vi "Details Display Dialog-MOD.vi"(0 "Source":string, 1 "Start":i32[](array[numeric]), 2 "Length":i32[](array[numeric]), 5 "Details":string="reason for problem", 7 "dialog type":T2, 9 "Error or Warning":bool, 11 "contname":string="Continue", 12 "stopname":string="Stop", 13 "okname":string="OK") -> (4 "STOP?":bool, 15 "stop event propagated":bool)   [LabVIEW 2013]
uses:
  <vilib>/Utility/error.llb/DialogTypeEnum.ctl
  <vilib>/Utility/error.llb/ErrWarn.ctl
  <vilib>/event_ctls.llb/eventvkey.ctl
panel:
  in  "truncated message":string="(source truncated)"
  in  "truncated & CH message":string="(source truncated; see Context Help window)"
  out "Source of Error":string
  out "scrollbar text":string
  in  "Test for size":string
  out "text":string
  out "Error or Warning Glyph":T1=TRUE
  in  "OK":bool
  in  "Stop":bool
  in  "Continue":bool
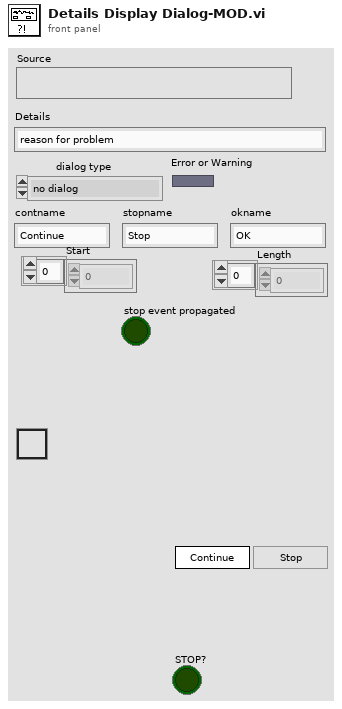
[diagram p1: front panel]
types:
  T1 = typedef "ErrWarn.ctl" = bool
  T2 = typedef "DialogTypeEnum.ctl" = enum16{"no dialog", "OK message", "continue or stop message", "auto error handling dialog", "OK message + warnings", "continue/stop + warnings"}
  T3 = typedef "eventvkey.ctl" = enum16{"ASCII", "Enter", "Return", "Shift", "Ctrl", "Alt", "Cmd", "Opt", "Caps", "NumLock", "Clear", "Break", "Up", "Down", "Left", "Right", "Insert", "Delete", "Home", "End", "PageUp", "PageDown", "Escape", "Help", "Pause", "ScrollLock", "F1", "F2", "F3", "F4", "F5", "F6", "F7", "F8", "F9", "F10", "F11", "F12", "F13", "F14", "F15", "F16", "F17", "F18", "F19", "F20", "F21", "F22", "F23", "F24", "Play", "VolumeUp", "VolumeDown", "Mute", "Two Byte Char"}
  T4 = typedef "LVRectTypeDef.ctl" = cluster{"Left":i16, "Top":i16, "Right":i16, "Bottom":i16}
  T5 = cluster{"Control":bool, "Shift":bool, "Key":string}
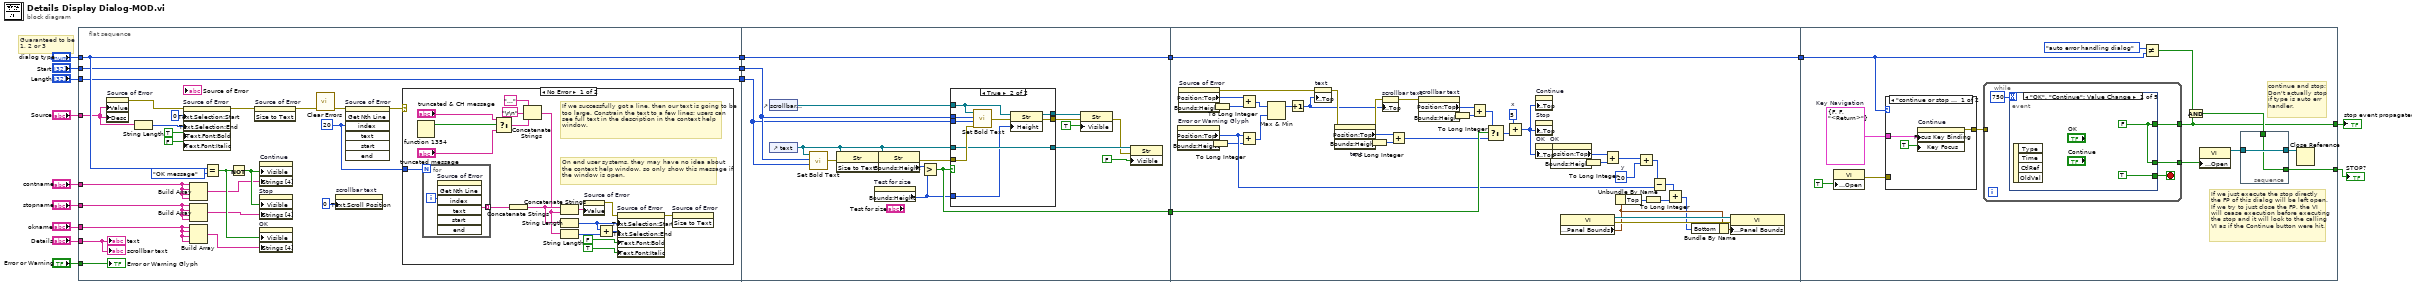
[diagram p0: block diagram]
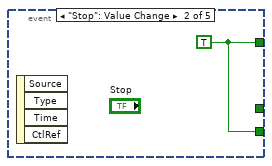
[diagram p4: hidden frame]
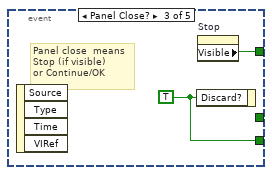
[diagram p5: hidden frame]
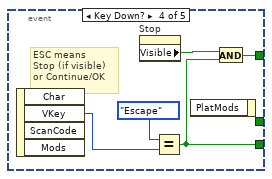
[diagram p6: hidden frame]
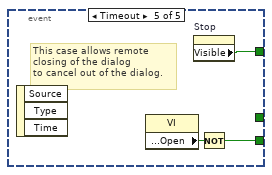
[diagram p7: hidden frame]
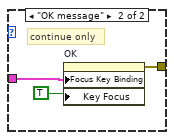
[diagram p8: hidden frame]
diagram:
  # "Guaranteed to be\n1, 2 or 3"
  n1 = flat-sequence {
    tunnel: [w26] -> w16
    tunnel: "dialog type" -> [w26]
    tunnel: "contname" -> [w25]
    tunnel: "stopname" -> [w24]
    tunnel: "okname" -> [w23]
    tunnel: "Source" -> [w18]
    tunnel: "Details" -> [w22]
    tunnel: "Error or Warning" -> [w21]
    tunnel: [w20] -> w5
    tunnel: [w19] -> w4
    tunnel: "Start" -> [w20]
    tunnel: "Length" -> [w19]
    tunnel: w16 -> [w66]
    tunnel: [w66] -> w15
    tunnel: [w72] -> w14
    tunnel: w5 -> [w65]
    tunnel: w4 -> [w64]
    tunnel: w15 -> [w99]
    tunnel: [w99] -> w13
    tunnel: w14 -> [w134]
    tunnel: [w136] -> w17
    tunnel: w13 -> [w138]
    tunnel: [w135] -> w1
    frame #0 {
      w33 = u32 20 ("index")
      n2 = property on="Source of Error" class="Str"("Value"=w18, "Desc"=w18) -> (error out=w32:errorcluster)  [unwired: 2 in, 1 out]
      n3 = String Length(string=w18) -> (length=w29:i32)
      n4 = property on="Source of Error" class="Str"(error in=w32, "Text.Selection:Start"=u32 0, "Text.Selection:End"=w29, "Text.Font:Bold"=TRUE, "Text.Font:Italic"=FALSE) -> (error out=w31:errorcluster)  [unwired: 1 in, 1 out]
      n5 = Build Array(w25, w25, w25, w25) -> (w41:string[])
      n6 = Build Array(w24, w24, w24, w24) -> (w40:string[])
      n7 = Build Array(w23, w23, w23, w23) -> (w39:string[])
      n8 = Equal?(x=w26, y=DialogTypeEnum."OK message" ("dialog type")) -> (x = y?=w43:bool)
      n9 = Not(x=w43) -> (.not. x?=w42:bool)
      n10 = invoke on="Source of Error" class="Str" method="Size to Text"(error in=w31) -> (error out=w36:errorcluster)  [unwired: 2 in, 2 out]
      n11 = property on="Continue" class="Bool"("Visible"=w42, "Strings [4]"=w41) -> ()  [unwired: 2 in, 2 out]
      n12 = property on="Stop" class="Bool"("Visible"=w42, "Strings [4]"=w40) -> ()  [unwired: 2 in, 2 out]
      n13 = property on="OK" class="Bool"("Visible"=w43, "Strings [4]"=w39) -> ()  [unwired: 2 in, 2 out]
      n14 = call <vilib>:"Clear Errors.vi"("error in (no error)"=w36) -> ("error out"=w35:errorcluster)  [unwired: 6 out]
      n15 = property on="scrollbar text" class="Str"("Text.Scroll Position"=u32 0) -> ()  [unwired: 2 in, 2 out]
      n16 = invoke on="Source of Error" class="Str" method="Get Nth Line"(error in=w35, "index"=w33) -> (error out=w34:errorcluster)  [unwired: 5 in, 6 out]
      n17 = case shown="No Error" w34 {
        tunnel: w33 -> [w61 _]
        frame No Error {
          # "If we successfully got a line, then our text is going to be too large. Constrain the text to a few lines; users can see full text in the description in the context help window."
          # "On end user systems, they may have no idea about\nthe context help window, so only show this message if\nthe window is open."
          n18 = fn#1354() -> (1:w51:bool)  [unwired: 1 out]
          n19 = for {
            N: w61 -> [_]
            tunnel: [w62] -> w59 mode=indexing
            i -> [w63]
            n20 = invoke on="Source of Error" class="Str" method="Get Nth Line"("index"=w63) -> ("text"=w62:string)  [unwired: 6 in, 6 out]
          }
          n21 = Select(t="truncated & CH message", s=w51, f="truncated message") -> (s? t:f=w48:string)
          n22 = Concatenate Strings(w59) -> (w58:string)
          n23 = Concatenate Strings("..." ("string"), "\r\n", w48) -> (w45:string)
          n24 = Concatenate Strings(w58, w45) -> (w60:string)
          n25 = String Length(string=w58) -> (length=w53:i32)
          n26 = String Length(string=w45) -> (length=w50:i32)
          n27 = property on="Source of Error" class="Str"("Value"=w60) -> (error out=w55:errorcluster)  [unwired: 2 in, 1 out]
          n28 = Add(x=w53, y=w50) -> (x+y=w52:i32)
          n29 = property on="Source of Error" class="Str"(error in=w55, "Text.Selection:Start"=w53, "Text.Selection:End"=w52, "Text.Font:Bold"=FALSE, "Text.Font:Italic"=TRUE) -> (error out=w54:errorcluster)  [unwired: 1 in, 1 out]
          n30 = invoke on="Source of Error" class="Str" method="Size to Text"(error in=w54) -> ()  [unwired: 2 in, 3 out]
        }
        frame Error {
          # "An error at this point means that there is no line to fetch. That's good. We do not want the text getting too large."
        }
      }
      "Error or Warning Glyph" <- w21
      "scrollbar text" <- w22
      "text" <- w22
    }
    frame #1 {
      n31 = control-ref of="scrollbar text"() -> (w75:refnum<vi>)
      n32 = control-ref of="text"() -> (w67:refnum<vi>)
      n33 = call <vilib>:"Set Bold Text.vi"("Length"=w64, "Start"=w65, "text"=w67) -> ("error out"=w70:errorcluster)  [unwired: 1 in, 2 out]
      n34 = invoke class="Str" method="Size to Text"(reference=w67, error in=w70) -> (error out=w71:errorcluster)  [unwired: 1 in, 2 out]
      n35 = property on="Test for size" class="Str"() -> ("Bounds:Height"=w69:u32)  [unwired: 2 in, 2 out]
      n36 = property class="Str"(reference=w67, error in=w71) -> (error out=w79:errorcluster, "Bounds:Height"=w80:u32)  [unwired: 1 out]
      n37 = Greater?(x=w80, y=w69) -> (0:w72:bool)
      n38 = case shown="True" w72 {
        tunnel: w79 -> [w83 w92]
        tunnel: w65 -> [_ w91]
        tunnel: w64 -> [_ w90]
        tunnel: [w83 w87] -> w68
        tunnel: w67 -> [w82 w89]
        tunnel: [w82 w84] -> w77
        tunnel: [w81 w89] -> w76
        tunnel: w75 -> [w81 w85]
        tunnel: w69 -> [_ w88]
        frame False {
        }
        frame True {
          n39 = call <vilib>:"Set Bold Text.vi"("error in"=w92, "Length"=w90, "Start"=w91, "text"=w85) -> ("error out"=w86:errorcluster)  [unwired: 2 out]
          n40 = property class="Str"(reference=w85, error in=w86, "Height"=w88) -> (reference out=w84:refnum<vi>, error out=w87:errorcluster)
        }
      }
      n41 = property class="Str"(reference=w77, error in=w68, "Visible"=TRUE ("Defer Panel Updates")) -> (error out=w73:errorcluster)  [unwired: 1 out]
      n42 = property class="Str"(reference=w76, error in=w73, "Visible"=FALSE ("Defer Panel Updates")) -> ()  [unwired: 2 out]
    }
    frame #2 {
      w120 = 20  # y
      w125 = 5  # x
      n43 = property on="Error or Warning Glyph" class="Bool"() -> ("Position:Top"=w115:i32, "Bounds:Height"=w131:u32)  [unwired: 2 in, 2 out]
      n44 = property on="Source of Error" class="Str"() -> (error out=w100:errorcluster, "Position:Top"=w102:i32, "Bounds:Height"=w101:u32)  [unwired: 2 in, 1 out]
      n45 = To Long Integer(number=w131) -> (32bit integer=w98:i32)
      n46 = To Long Integer(number=w101) -> (32bit integer=w97:i32)
      n47 = Add(x=w102, y=w97) -> (x+y=w133:i32)
      n48 = Add(x=w115, y=w98) -> (x+y=w132:i32)
      n49 = Max & Min(x=w133, y=w132) -> (max(x,y)=w130:i32)  [unwired: 1 out]
      n50 = Increment(x=w130) -> (x+1=w108:i32)
      n51 = property on="text" class="Str"(error in=w100, "Position:Top"=w108) -> (error out=w110:errorcluster)  [unwired: 1 in, 1 out]
      n52 = property on="text" class="Str"(error in=w110) -> (error out=w109:errorcluster, "Position:Top"=w107:i32, "Bounds:Height"=w106:u32)  [unwired: 1 in, 1 out]
      n53 = To Long Integer(number=w106) -> (32bit integer=w96:i32)
      n54 = property on="scrollbar text" class="Str"(error in=w109, "Position:Top"=w108) -> (error out=w129:errorcluster)  [unwired: 1 in, 1 out]
      n55 = Add(x=w107, y=w96) -> (x+y=w104:i32)
      n56 = property on="scrollbar text" class="Str"(error in=w129) -> ("Position:Top"=w128:i32, "Bounds:Height"=w127:u32)  [unwired: 1 in, 2 out]
      n57 = To Long Integer(number=w127) -> (32bit integer=w95:i32)
      n58 = Add(x=w128, y=w95) -> (x+y=w105:i32)
      n59 = Select(t=w105, s=w134, f=w104) -> (s? t:f=w103:i32)
      n60 = Add(x=w125, y=w103) -> (x+y=w126:i32)
      n61 = property on="Continue" class="Bool"("Position:Top"=w126) -> ()  [unwired: 2 in, 2 out]
      n62 = property on="Stop" class="Bool"("Position:Top"=w126) -> ()  [unwired: 2 in, 2 out]
      n63 = property on="OK" class="Bool"("Position:Top"=w126) -> (error out=w124:errorcluster)  [unwired: 2 in, 1 out]
      n64 = property on="OK" class="Bool"(error in=w124) -> ("Position:Top"=w122:i32, "Bounds:Height"=w123:u32)  [unwired: 1 in, 2 out]
      n65 = property class="VI"() -> (reference out=w117:refnum<vi>, error out=w118:errorcluster, "Front Panel Window:Panel Bounds"=w114:T4)  [unwired: 2 in]
      n66 = To Long Integer(number=w123) -> (32bit integer=w94:i32)
      n67 = Add(x=w122, y=w94) -> (x+y=w121:i32)
      n68 = Unbundle By Name(w114) -> ("Top"=w112:i16)
      n69 = Add(x=w121, y=w120) -> (x+y=w116:i32)
      n70 = To Long Integer(number=w112) -> (32bit integer=w93:i32)
      n71 = Subtract(x=w116, y=w115) -> (x-y=w113:i32)
      n72 = Add(x=w113, y=w93) -> (x+y=w111:i32)
      n73 = Bundle By Name(cluster=w114, "Bottom"=w111) -> (w119:T4)
      n74 = property class="VI"(reference=w117, error in=w118, "Front Panel Window:Panel Bounds"=w119) -> ()  [unwired: 2 out]
    }
    frame #3 {
      w147 = T5 {"Control"=FALSE, "Shift"=FALSE, "Key"="<Return>"}  # Key Navigation
      # "If we just execute the stop directly\nthe FP of this dialog will be left open.\nIf we try to just close the FP, the VI\nwill cease execution before executing\nthe stop and it will look to the calling\nVI as if the Continue button were hit."
      # "continue and stop;\nDon't actually stop\nif type is auto err\nhandler."
      n75 = property class="VI"("Front Panel Window:Open"=TRUE) -> (error out=w146:errorcluster)  [unwired: 2 in, 1 out]
      n76 = case shown="\"continue or stop message\", Default" w138 {
        tunnel: w147 -> [w169 w172]
        tunnel: w146 -> [_ _]
        tunnel: [w167 w170] -> w144
        frame "continue or stop message", Default {
          n77 = property on="Continue" class="Bool"("Focus Key Binding"=w169, "Key Focus"=TRUE) -> (error out=w167:errorcluster)  [unwired: 2 in, 1 out]
        }
        frame "OK message" {
          # "continue only"
          n78 = property on="OK" class="Bool"("Focus Key Binding"=w172, "Key Focus"=TRUE) -> (error out=w170:errorcluster)  [unwired: 2 in, 1 out]
        }
      }
      n79 = while {
        tunnel: w144 -> [_]
        tunnel: [w152] -> w136
        tunnel: [w151] -> w137
        stop <- w153 stop-if-true
        n80 = event shown="[0] \"OK\", \"Continue\": Value Change" {
          selector: _ -> [_ _ _ _ _]
          dyn-events: _ -> [_ _ _ _ _]
          timeout: 750 -> [_ _ _ _ _]
          tunnel: [TRUE ("Stop") w156 w158 w159 w164] -> w153
          tunnel: [w155 w156 w157 w162 w166] -> w152
          tunnel: [w155 _ _ _ _] -> w151
          event "OK", "Continue": Value Change {
            w155 = FALSE ("Stop")
            n81 = event-data() -> ()  [unwired: 5 out]
          }
          event "Stop": Value Change {
            w156 = TRUE
            n82 = event-data() -> ()  [unwired: 5 out]
          }
          event Panel Close? {
            w158 = TRUE ("Discard?")
            # "Panel close  means\nStop (if visible)\nor Continue/OK"
            n83 = event-data() -> ()  [unwired: 5 out]
            n84 = event-data("Discard?"=w158) -> ()  [unwired: 1 in, 1 out]
            n85 = property on="Stop" class="Bool"() -> ("Visible"=w157:bool)  [unwired: 2 in, 2 out]
          }
          event Key Down? {
            # "ESC means\nStop (if visible)\nor Continue/OK"
            n86 = event-data() -> ("VKey"=w161:T3)  [unwired: 4 out]
            n87 = property on="Stop" class="Bool"() -> ("Visible"=w163:bool)  [unwired: 2 in, 2 out]
            n88 = Equal?(x=eventvkey."Escape", y=w161) -> (x = y?=w159:bool)
            n89 = event-data() -> ()  [unwired: 1 in, 2 out]
            n90 = And(x=w163, y=w159) -> (x .and. y?=w162:bool)
          }
          event Timeout {
            # "This case allows remote\nclosing of the dialog\nto cancel out of the dialog."
            n91 = event-data() -> ()  [unwired: 4 out]
            n92 = property class="VI"() -> ("Front Panel Window:Open"=w165:bool)  [unwired: 2 in, 2 out]
            n93 = property on="Stop" class="Bool"() -> ("Visible"=w166:bool)  [unwired: 2 in, 2 out]
            n94 = Not(x=w165) -> (.not. x?=w164:bool)
          }
        }
      }
      n95 = Not Equal?(x=DialogTypeEnum."auto error handling dialog" ("dialog type"), y=w138) -> (x != y?=w143:bool)
      n96 = And(x=w143, y=w136) -> (x .and. y?=w142:bool)
      n97 = property class="VI"("Front Panel Window:Open"=w137) -> (reference out=w140:refnum<vi>)  [unwired: 2 in, 1 out]
      n98 = stacked-sequence {
        tunnel: w140 -> [w149]
        tunnel: w142 -> [w148]
        tunnel: [w149] -> w141
        tunnel: [w148] -> w135
        frame #0 {
        }
      }
      n99 = Close Reference(reference=w141) -> ()  [unwired: 1 in, 1 out]
    }
  }
  "stop event propagated" <- w17
  "STOP?" <- w1
